vi "Diagram - Connect Tunnel with Wire 2.vi"(8 "error in (no error)":errorcluster, 9 "Wire Indexs":i32[](array[numeric]), 10 "Front Tunnels":refnum<vi>[](array[refnum]), 11 "Diagram in":refnum<vi>) -> (0 "error out":errorcluster, 2 "Array out":i32[](array[numeric]), 3 "Diagram out":refnum<vi>)   [LabVIEW 2017, in "csmHelper-Diagram.lvlib"]
doc: "-- <b>输入控件</b> --\n- <b>error in (no error)</b>:\n- <B>error in</B> can accept error information wired from VIs previously called. Use this information to decide if any functionality should be bypassed in the event of errors from other VIs.\n\nRight-click the <B>error in</B> control on the front panel and select <B>Explain Error</B> or <B>Explain Warning</B> from the shortcut menu for more information about the error.\n- <b>Wire Indexs</b>:\n\n- <b>Front Tunnels</b>:\n\n- <b>Diagram in</b>:\n\n\n-- <b>输出控件</b> --\n- <b>error out</b>:\n- <B>error in</B> can accept error information wired from VIs previously called. Use this information to decide if any functionality should be bypassed in the event of errors from other VIs.\n\nRight-click the <B>error in</B> control on the front panel and select <B>Explain Error</B> or <B>Explain Warning</B> from the shortcut menu for more information about the error.\n- <b>Array out</b>:\n\n- <b>Diagram out</b>:"
uses:
  csmHelper-Diagram.lvlib
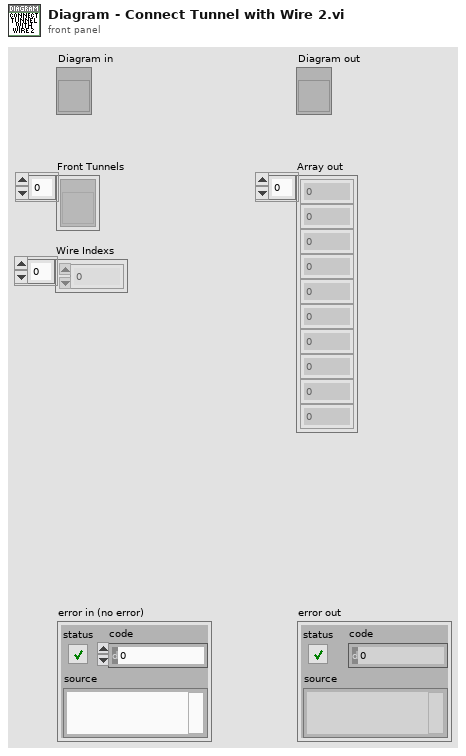
[diagram p1: front panel]
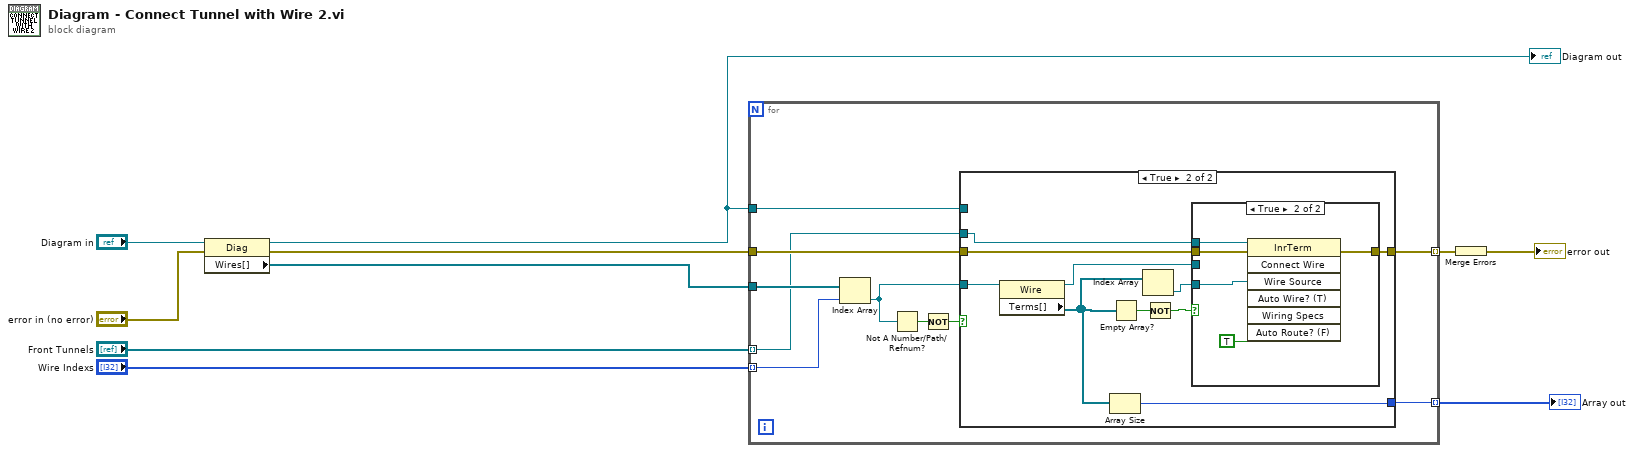
[diagram p0: block diagram]
diagram:
  n1 = property on="Property Node" class="Diag"(reference="Diagram in", error in="error in (no error)") -> (reference out=w8:refnum<vi>, error out=w10:errorcluster, "Wires[]"=w1:refnum<vi>[])
  "Diagram out" <- w8
  n2 = for {
    tunnel: w1 -> [w18]
    tunnel: "Wire Indexs" -> [w17] mode=indexing
    tunnel: "Front Tunnels" -> [w16] mode=indexing
    tunnel: w10 -> [w20]
    tunnel: [w19] -> w2 mode=indexing
    tunnel: [w13] -> w6 mode=indexing
    tunnel: w8 -> [w12]
    n3 = Index Array(array=w18, index=w17) -> (element=w14:refnum<vi>)
    n4 = Not A Number/Path/Refnum?(number/path/refnum=w14) -> (NaN/Path/Refnum?=w11:bool)
    n5 = Not(x=w11) -> (.not. x?=w15:bool)
    n6 = case shown="True" w15 {
      tunnel: w20 -> [w21 w31]
      tunnel: [w21 w30] -> w19
      tunnel: w14 -> [_ w29]
      tunnel: w16 -> [_ w27]
      tunnel: [_ w28] -> w13
      tunnel: w12 -> [_ _]
      frame False {
      }
      frame True {
        n7 = property class="Wire"(reference=w29) -> (reference out=w23:refnum<vi>, "Terms[]"=w25:refnum<vi>[])  [unwired: 1 in, 1 out]
        n8 = Array Size(array=w25) -> (size(s)=w28:i32)
        n9 = Empty Array?(array=w25) -> (empty?=w22:bool)
        n10 = Index Array(array=w25) -> (element=w24:refnum<vi>)  [unwired: 1 in]
        n11 = Not(x=w22) -> (.not. x?=w26:bool)
        n12 = case shown="True" w26 {
          tunnel: w31 -> [w32 w37]
          tunnel: [w32 w36] -> w30
          tunnel: w27 -> [_ w34]
          tunnel: w24 -> [_ w33]
          tunnel: w23 -> [_ _]
          frame False {
          }
          frame True {
            n13 = invoke class="InrTerm" method="Connect Wire"(reference=w34, error in=w37, "Wire Source"=w33, "Auto Route? (F)"=TRUE) -> (error out=w36:errorcluster)  [unwired: 3 in, 6 out]
          }
        }
      }
    }
  }
  "Array out" <- w6
  n14 = Merge Errors(w2) -> (→"error out":errorcluster)
